vi "GMT Delta.vi"() -> (0 "GMT Delta in seconds":dbl format="%.2f")   [LabVIEW 2009, in "Tools_String.lvlib"]
doc: "Returns this time zone's offset in seconds with respect to GMT."
uses:
  Tools_String.lvlib
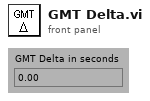
[diagram p1: front panel]
types:
  T1 = cluster{"second":i32, "minute":i32, "hour":i32, "day of month":i32, "month":i32, "year":i32, "day of week":i32, "day of year":i32, "is DST":i32}
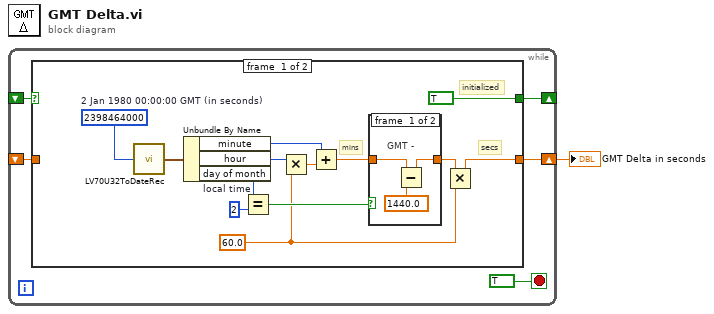
[diagram p0: block diagram]
diagram:
  n1 = while {
    shift-left: _ -> [w5]
    shift-right: [w4] -> _
    shift-left: _ -> [w3]
    shift-right: [w6] -> w1
    stop <- TRUE stop-if-true
    n2 = case shown="False" w5 {
      selector: w5 -> [_ w25]
      tunnel: [w12 w24] -> w6
      tunnel: [TRUE w25] -> w4
      tunnel: w3 -> [_ w24]
      frame #0 {
        w14 = u32 2398464000  # 2 Jan 1980 00:00:00 GMT (in seconds)
        w13 = 60.0
        # "initialized"
        # "mins"
        # "secs"
        n3 = call <vilib>:"LV70U32ToDateRec.vi"("Time"=w14) -> ("date time rec"=w19:T1)
        n4 = Unbundle By Name "local time"(w19) -> ("minute"=w8:i32, "hour"=w10:i32, "day of month"=w18:i32)
        n5 = Equal?(x=w18, y=2) -> (x = y?=w16:bool)
        n6 = Multiply(x=w10, y=w13) -> (x*y=w9:dbl)
        n7 = Add(x=w8, y=w9) -> (x+y=w7:dbl)
        n8 = case shown="False" w16 {
          tunnel: [w22 w23] -> w11
          tunnel: w7 -> [w20 w23]
          frame #0 {
            # "GMT -"
            n9 = Subtract(x=w20, y=1440.0) -> (x-y=w22:dbl)
          }
          frame #1 {
            # "GMT +"
          }
        }
        n10 = Multiply(x=w11, y=w13) -> (x*y=w12:dbl)
      }
      frame #1 {
        # "already initialized"
      }
    }
  }
  "GMT Delta in seconds" <- w1
